vi "99乘法表.vi"() -> ()   [LabVIEW 2019]
panel:
  out "Array":dbl[][](array[numeric])
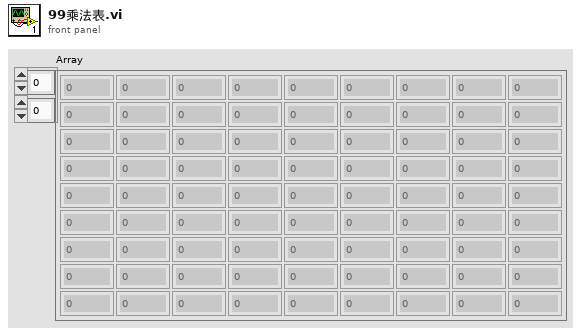
[diagram p1: front panel]
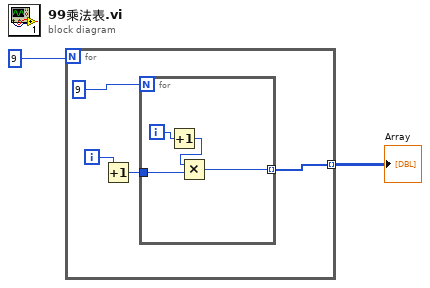
[diagram p0: block diagram]
diagram:
  n1 = for {
    N: 9 -> [_]
    tunnel: [w5] -> w1 mode=indexing
    i -> [w4]
    n2 = Increment(x=w4) -> (x+1=w3:i32)
    n3 = for {
      N: 9 -> [_]
      tunnel: [w10] -> w5 mode=indexing
      tunnel: w3 -> [w7]
      i -> [w9]
      n4 = Increment(x=w9) -> (x+1=w8:i32)
      n5 = Multiply(x=w8, y=w7) -> (x*y=w10:i32)
    }
  }
  "Array" <- w1
